vi "Append Report Text (num).vi"(0 "report in":refnum<class "NI_Standard Report.lvclass">, 1 "MS Office parameters":T1, 2 "format string (%.3f)":string="%.3f", 7 "text":dbl format="%.2f", 9 "append on new line? (F)":bool, 11 "error in (no error)":errorcluster) -> (4 "report out":refnum<class "NI_Standard Report.lvclass">, 8 "start out (Word)":i32, 10 "end out (Word)":i32, 15 "error out":errorcluster)   [LabVIEW 2017, in "NI_Standard Report.lvclass"]
doc: "Appends text to the selected report."
uses:
  <vilib>/Utility/NIReport.llb/Standard Report/NI_Standard Report.lvclass
  <vilib>/Utility/NIReport.llb/Standard Report/NI_Standard Report.lvclass/NI_Standard Report.ctl
  <vilib>/Utility/NIReport.llb/NI_ReportGenerationCore.lvlib
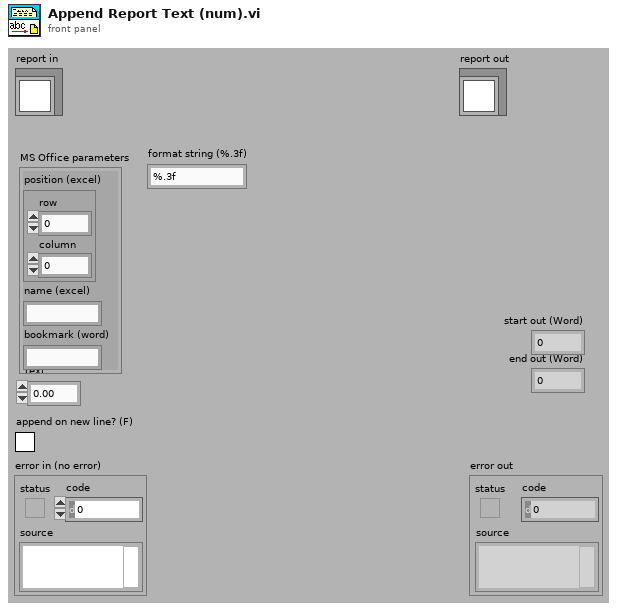
[diagram p1: front panel]
types:
  T1 = cluster{"position (excel)":cluster{"row":i32, "column":i32}, "name (excel)":string, "bookmark (word)":string}
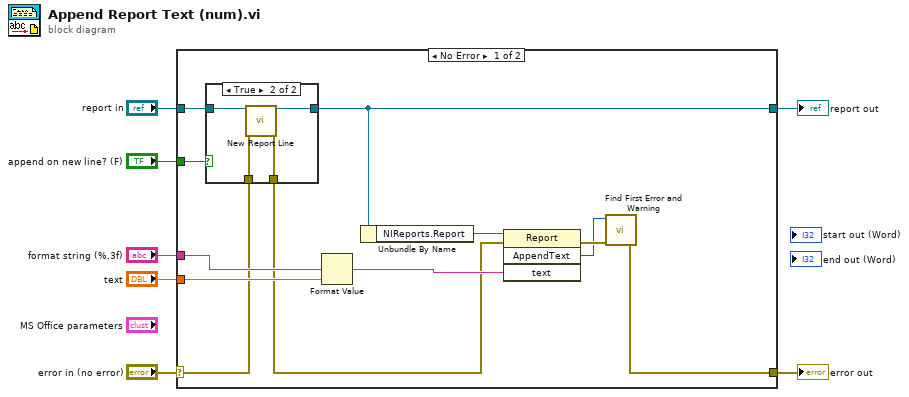
[diagram p0: block diagram]
diagram:
  n1 = case shown="No Error" "error in (no error)" {
    selector: "error in (no error)" -> [w9 w27]
    tunnel: [w10 w27] -> w6
    tunnel: [w13 w26] -> w4
    tunnel: "report in" -> [w19 w26]
    tunnel: "append on new line? (F)" -> [w18 _]
    tunnel: "text" -> [w15 _]
    tunnel: "format string (%.3f)" -> [w14 _]
    frame No Error {
      n2 = case shown="True" w18 {
        tunnel: w19 -> [w21 w25]
        tunnel: [w21 w24] -> w13
        tunnel: w9 -> [w20 w23]
        tunnel: [w20 w22] -> w8
        frame False {
        }
        frame True {
          n3 = call-dynamic "New Report Line.vi"("report in"=w25, "error in (no error)"=w23) -> ("report out"=w24:refnum<class "NI_Standard Report.lvclass">, "error out"=w22:errorcluster)  [unwired: 1 in, 11 out]
        }
      }
      n4 = Format Value(format string=w14, value (0)=w15) -> (output string=w16:string)  [unwired: 1 out]
      n5 = Unbundle By Name(w13) -> ("NIReports.Report"=w17:refnum<k7>)
      n6 = invoke class="Report" method="AppendText"(reference=w17, error in=w8, "text"=w16) -> (error out=w12:errorcluster, "AppendText"=w11:i32)  [unwired: 1 in, 2 out]
      n7 = call <vilib>:"Find First Error and Warning.vi"("error in (no error)"=w12, "error code"=w11) -> ("error out"=w10:errorcluster)  [unwired: 1 in, 4 out]
    }
    frame Error {
    }
  }
  "error out" <- w6
  "report out" <- w4
